vi "Param Global.vi"(7 "Operate":T2=enum."Read", 8 "error in (no error)":errorcluster caption="Error In", 9 "Param In":T1={"RH(%)"={"DS"={"阳极露点温度_DS"="TIRC101_PV", "阳极出口温度_DS"="TIR104_PV", "阴极露点温度_DS"="TIRC301_PV", "阴极出口温度_DS"="TIRC301_PV", "阳极相对湿度_DS"="SY_RH_An", "阴极相对湿度_DS"="SY_RH_Ca", "阳极露点温度设置_DS"="TIRC101_PV", "阳极出口温度设置_DS"="TIR104_PV", "阴极露点温度设置_DS"="TIRC301_PV", "阴极出口温度设置_DS"="TIRC301_PV"}, "Value"={"阳极露点温度_PV"=0.0, "阳极出口温度_PV"=0.0, "阴极露点温度_PV"=0.0, "阴极出口温度_PV"=0.0, "阳极相对湿度_SY"=0.0, "阴极相对湿度_SY"=0.0, "阳极露点温度设置_SV"=0.0, "阳极出口温度设置_SV"=0.0, "阴极露点温度设置_SV"=0.0, "阴极出口温度设置_SV"=0.0}}, "WEB"={"DS"={"自动模式(M0A1)_DS"="AUTO_MODE", "设备运行_DS"="DEVICE_STATE", "工步号_DS"="DEVICE_STATE", "运行模式_DS"="DEVICE_STATE"}, "Value"={"自动模式(M0A1)_PV"=FALSE, "设备运行_PV"=FALSE, "工步号_PV"=0.0, "运行模式_PV"=FALSE}}, "ELD"={"DS"={"负载电压设置_DS"="EL_V_SET", "负载电流设置_DS"="EL_A_SET", "负载功率设置_DS"="EL_P_SET", "负载模式设置_DS"="EL_MODE", "错误代码_DS"="EL_ERROR", "负载电压_DS"="EL_V", "负载电流_DS"="EL_A", "负载功率_DS"="EL_P", "负载输出使能_DS"="EL_INPUT", "负载连接_DS"="ELD", "负载升压_DS"="SY_Load_Rise_Volt", "负载升流_DS"="SY_Load_Rise_Curr", "负载升功率_DS"="SY_Load_Rise_Power", "负载降压_DS"="SY_Load_Drop_Volt", "负载降流_DS"="SY_Load_Drop_Curr", "负载降功率_DS"="SY_Load_Drop_Power", "电流密度_DS"="Density_A_SV", "功率密度_DS"="Density_P_SV"}, "Value"={"负载电压设置_SV"=0.0, "负载电流设置_SV"=0.0, "负载功率设置_SV"=0.0, "负载模式设置_SV"="", "错误代码_PV"="", "负载电压_PV"=0.0, "负载电流_PV"=0.0, "负载功率_PV"=0.0, "负载输出使能_SV"=FALSE, "负载连接_SY"=FALSE, "负载升压_SV"=0.0, "负载升流_SV"=0.0, "负载升功率_SV"=0.0, "负载降压_SV"=0.0, "负载降流_SV"=0.0, "负载降功率_SV"=0.0, "电流密度_SV"=0.0, "功率密度_SV"=0.0}}, "SY"={"DS"={"总报警_DS"="SY_Totol_Warning", "WEB连接_DS"="SY_Web_Con", "计量比功能_DS"="SY_Measurung_Ratio", "PLC连接_DS"="SY_Measurung_Ratio", "H2计量比功能_DS"="SY_Measurung_Ratio", "Air计量比功能_DS"="SY_Measurung_Ratio", "PLC失联报警_DS"="SY_Measurung_Ratio"}, "Value"={"总报警_PV"=FALSE, "WEB连接_PV"=FALSE, "计量比功能_SV"=FALSE, "PLC连接_SV"=FALSE, "H2计量比功能_SV"=FALSE, "Air计量比功能_SV"=FALSE, "PLC失联报警_SV"=FALSE}}, "PLC"={"DS"={"PLC急停_DS"="HMI_Estop_SV", "PLC连接_DS"="PLC", "下位机心跳值_DS"="PLC", "上位机心跳值_DS"="HMI_AlarmWord_SV", "上位机报警等级字_DS"="HMI_AlarmWord_SV", "负载可卸载_DS"="HMI_AlarmWord_SV"}, "Value"={"PLC急停_PV"=FALSE, "PLC连接_PV"=FALSE, "下位机心跳值_PV"=0.0, "上位机心跳值_SV"=0.0, "上位机报警等级字_SV"=0.0, "负载可卸载_SV"=FALSE}}, "Bool Control"={"DS"={"维护模式_DS"="WorkMode_SV", "阳极氮气吹扫_DS"="An_Purge_SV", "阴极氮气吹扫_DS"="Ca_Purge_SV", "阳极脉冲使能_DS"="An_Pulse_EN_SV", "准备好使能_DS"="DEVICE_READY", "阳极干湿气切换_DS"="An_GasMode_SV", "阴极干湿气切换_DS"="Ca_GasMode_SV", "自动/手动模式_DS"="AUTO_MODE", "入口背压_DS"="Stack_PreMode_SV", "手动卸载_DS"="HMI_Stack_OFF_SV", "软急停_DS"="HMI_Estop_SV", "负载连接_DS"="ELoad_EN_SV", "PLC故障复位_DS"="PLC_Alarm_Reset_SV", "蜂鸣器屏蔽_DS"="BuzzerShield_SV"}, "Value"={"维护模式_SV"=FALSE, "阳极氮气吹扫_SV"=FALSE, "阴极氮气吹扫_SV"=FALSE, "阳极脉冲使能_SV"=FALSE, "准备好使能_SV"=FALSE, "阳极干湿气切换_SV"=FALSE, "阴极干湿气切换_SV"=FALSE, "自动/手动模式_SV"=FALSE, "入口背压_SV"=FALSE, "手动卸载_SV"=FALSE, "软急停_SV"=FALSE, "负载连接_SV"=FALSE, "PLC故障复位_SV"=FALSE, "蜂鸣器屏蔽_SV"=FALSE}}, "Stoich"={"DS"={"H2初始流量_DS"="SY_Activation_Area", "Ait初始流量_DS"="SY_Pieces", "H2侧系数_DS"="SY_Activation_Area", "Air侧系数_DS"="SY_Pieces", "H2计量比_DS"="SY_Stoich_H2", "Air计量比_DS"="SY_Stoich_Air", "时间间隔_DS"="SY_Stoich_Interval", "H2计算气量_DS"="SY_Stoich_H2Flow", "Air计算气量_DS"="SY_Stoich_AirFlow", "H2流量_DS"="SY_Stoich_H2Flow", "Air流量_DS"="SY_Stoich_AirFlow"}, "Value"={"H2初始流量_SV"=0.0, "Ait初始流量_SV"=0.0, "H2侧系数_SV"=0.0, "Air侧系数_SV"=0.0, "H2计量比_SV"=0.0, "Air计量比_SV"=0.0, "时间间隔_SV"=0.0, "H2计算气量_SV"=0.0, "Air计算气量_SV"=0.0, "H2流量_DS"=0.0, "Air流量_DS"=0.0}}, "PLC Need"=[{"Name"="电堆电流_SV", "Identifier"="Stack_I_A_SV", "Source"="EL_A", "Value"=""}], "CVM"={"DS"={"活化面积_DS"="SY_Activation_Area", "开路电压_DS"="SY_OCV_Value", "单体总片数_DS"="SY_Pieces", "单体显示片数_DS"="SY_Pieces_Dis", "起始编号_DS"="SY_Starting_Number", "最大值"="SY_Activation_Area", "最大值编号_DS"="SY_OCV_Value", "最小值_DS"="SY_Pieces", "最小值编号_DS"="SY_Pieces_Dis", "选区合计电压_DS"="SY_Starting_Number", "平均值_DS"="SY_Pieces_Dis", "离均差_DS"="SY_Starting_Number"}, "Value"={"活化面积_SV"=0.0, "开路电压_SV"=0.0, "单体片数_SV"=0.0, "单体显示片数_SV"=0.0, "起始编号_SV"=0.0, "最大值_SV"=0.0, "最大值编号_SV"=0.0, "最小值_SV"=0.0, "最小值编号_SV"=0.0, "选区合计电压_SV"=0.0, "平均值_SV"=0.0, "离均差_SV"=0.0}}}, 11 "Project":string) -> (0 "error out":errorcluster caption="Error Out", 3 "Param Out":T1={"RH(%)"={"DS"={"阳极露点温度_DS"="TIRC101_PV", "阳极出口温度_DS"="TIR104_PV", "阴极露点温度_DS"="TIRC301_PV", "阴极出口温度_DS"="TIRC301_PV", "阳极相对湿度_DS"="SY_RH_An", "阴极相对湿度_DS"="SY_RH_Ca", "阳极露点温度设置_DS"="TIRC101_PV", "阳极出口温度设置_DS"="TIR104_PV", "阴极露点温度设置_DS"="TIRC301_PV", "阴极出口温度设置_DS"="TIRC301_PV"}, "Value"={"阳极露点温度_PV"=0.0, "阳极出口温度_PV"=0.0, "阴极露点温度_PV"=0.0, "阴极出口温度_PV"=0.0, "阳极相对湿度_SY"=0.0, "阴极相对湿度_SY"=0.0, "阳极露点温度设置_SV"=0.0, "阳极出口温度设置_SV"=0.0, "阴极露点温度设置_SV"=0.0, "阴极出口温度设置_SV"=0.0}}, "WEB"={"DS"={"自动模式(M0A1)_DS"="AUTO_MODE", "设备运行_DS"="DEVICE_STATE", "工步号_DS"="DEVICE_STATE", "运行模式_DS"="DEVICE_STATE"}, "Value"={"自动模式(M0A1)_PV"=FALSE, "设备运行_PV"=FALSE, "工步号_PV"=0.0, "运行模式_PV"=FALSE}}, "ELD"={"DS"={"负载电压设置_DS"="EL_V_SET", "负载电流设置_DS"="EL_A_SET", "负载功率设置_DS"="EL_P_SET", "负载模式设置_DS"="EL_MODE", "错误代码_DS"="EL_ERROR", "负载电压_DS"="EL_V", "负载电流_DS"="EL_A", "负载功率_DS"="EL_P", "负载输出使能_DS"="EL_INPUT", "负载连接_DS"="ELD", "负载升压_DS"="SY_Load_Rise_Volt", "负载升流_DS"="SY_Load_Rise_Curr", "负载升功率_DS"="SY_Load_Rise_Power", "负载降压_DS"="SY_Load_Drop_Volt", "负载降流_DS"="SY_Load_Drop_Curr", "负载降功率_DS"="SY_Load_Drop_Power", "电流密度_DS"="Density_A_SV", "功率密度_DS"="Density_P_SV"}, "Value"={"负载电压设置_SV"=0.0, "负载电流设置_SV"=0.0, "负载功率设置_SV"=0.0, "负载模式设置_SV"="", "错误代码_PV"="", "负载电压_PV"=0.0, "负载电流_PV"=0.0, "负载功率_PV"=0.0, "负载输出使能_SV"=FALSE, "负载连接_SY"=FALSE, "负载升压_SV"=0.0, "负载升流_SV"=0.0, "负载升功率_SV"=0.0, "负载降压_SV"=0.0, "负载降流_SV"=0.0, "负载降功率_SV"=0.0, "电流密度_SV"=0.0, "功率密度_SV"=0.0}}, "SY"={"DS"={"总报警_DS"="SY_Totol_Warning", "WEB连接_DS"="SY_Web_Con", "计量比功能_DS"="SY_Measurung_Ratio", "PLC连接_DS"="SY_Measurung_Ratio", "H2计量比功能_DS"="SY_Measurung_Ratio", "Air计量比功能_DS"="SY_Measurung_Ratio", "PLC失联报警_DS"="SY_Measurung_Ratio"}, "Value"={"总报警_PV"=FALSE, "WEB连接_PV"=FALSE, "计量比功能_SV"=FALSE, "PLC连接_SV"=FALSE, "H2计量比功能_SV"=FALSE, "Air计量比功能_SV"=FALSE, "PLC失联报警_SV"=FALSE}}, "PLC"={"DS"={"PLC急停_DS"="HMI_Estop_SV", "PLC连接_DS"="PLC", "下位机心跳值_DS"="PLC", "上位机心跳值_DS"="HMI_AlarmWord_SV", "上位机报警等级字_DS"="HMI_AlarmWord_SV", "负载可卸载_DS"="HMI_AlarmWord_SV"}, "Value"={"PLC急停_PV"=FALSE, "PLC连接_PV"=FALSE, "下位机心跳值_PV"=0.0, "上位机心跳值_SV"=0.0, "上位机报警等级字_SV"=0.0, "负载可卸载_SV"=FALSE}}, "Bool Control"={"DS"={"维护模式_DS"="WorkMode_SV", "阳极氮气吹扫_DS"="An_Purge_SV", "阴极氮气吹扫_DS"="Ca_Purge_SV", "阳极脉冲使能_DS"="An_Pulse_EN_SV", "准备好使能_DS"="DEVICE_READY", "阳极干湿气切换_DS"="An_GasMode_SV", "阴极干湿气切换_DS"="Ca_GasMode_SV", "自动/手动模式_DS"="AUTO_MODE", "入口背压_DS"="Stack_PreMode_SV", "手动卸载_DS"="HMI_Stack_OFF_SV", "软急停_DS"="HMI_Estop_SV", "负载连接_DS"="ELoad_EN_SV", "PLC故障复位_DS"="PLC_Alarm_Reset_SV", "蜂鸣器屏蔽_DS"="BuzzerShield_SV"}, "Value"={"维护模式_SV"=FALSE, "阳极氮气吹扫_SV"=FALSE, "阴极氮气吹扫_SV"=FALSE, "阳极脉冲使能_SV"=FALSE, "准备好使能_SV"=FALSE, "阳极干湿气切换_SV"=FALSE, "阴极干湿气切换_SV"=FALSE, "自动/手动模式_SV"=FALSE, "入口背压_SV"=FALSE, "手动卸载_SV"=FALSE, "软急停_SV"=FALSE, "负载连接_SV"=FALSE, "PLC故障复位_SV"=FALSE, "蜂鸣器屏蔽_SV"=FALSE}}, "Stoich"={"DS"={"H2初始流量_DS"="SY_Activation_Area", "Ait初始流量_DS"="SY_Pieces", "H2侧系数_DS"="SY_Activation_Area", "Air侧系数_DS"="SY_Pieces", "H2计量比_DS"="SY_Stoich_H2", "Air计量比_DS"="SY_Stoich_Air", "时间间隔_DS"="SY_Stoich_Interval", "H2计算气量_DS"="SY_Stoich_H2Flow", "Air计算气量_DS"="SY_Stoich_AirFlow", "H2流量_DS"="SY_Stoich_H2Flow", "Air流量_DS"="SY_Stoich_AirFlow"}, "Value"={"H2初始流量_SV"=0.0, "Ait初始流量_SV"=0.0, "H2侧系数_SV"=0.0, "Air侧系数_SV"=0.0, "H2计量比_SV"=0.0, "Air计量比_SV"=0.0, "时间间隔_SV"=0.0, "H2计算气量_SV"=0.0, "Air计算气量_SV"=0.0, "H2流量_DS"=0.0, "Air流量_DS"=0.0}}, "PLC Need"=[{"Name"="电堆电流_SV", "Identifier"="Stack_I_A_SV", "Source"="EL_A", "Value"=""}], "CVM"={"DS"={"活化面积_DS"="SY_Activation_Area", "开路电压_DS"="SY_OCV_Value", "单体总片数_DS"="SY_Pieces", "单体显示片数_DS"="SY_Pieces_Dis", "起始编号_DS"="SY_Starting_Number", "最大值"="SY_Activation_Area", "最大值编号_DS"="SY_OCV_Value", "最小值_DS"="SY_Pieces", "最小值编号_DS"="SY_Pieces_Dis", "选区合计电压_DS"="SY_Starting_Number", "平均值_DS"="SY_Pieces_Dis", "离均差_DS"="SY_Starting_Number"}, "Value"={"活化面积_SV"=0.0, "开路电压_SV"=0.0, "单体片数_SV"=0.0, "单体显示片数_SV"=0.0, "起始编号_SV"=0.0, "最大值_SV"=0.0, "最大值编号_SV"=0.0, "最小值_SV"=0.0, "最小值编号_SV"=0.0, "选区合计电压_SV"=0.0, "平均值_SV"=0.0, "离均差_SV"=0.0}}})   [LabVIEW 2020]
uses:
  Data Global/Data Global Mode.ctl
  0007 Controls/SY_Parameter.ctl
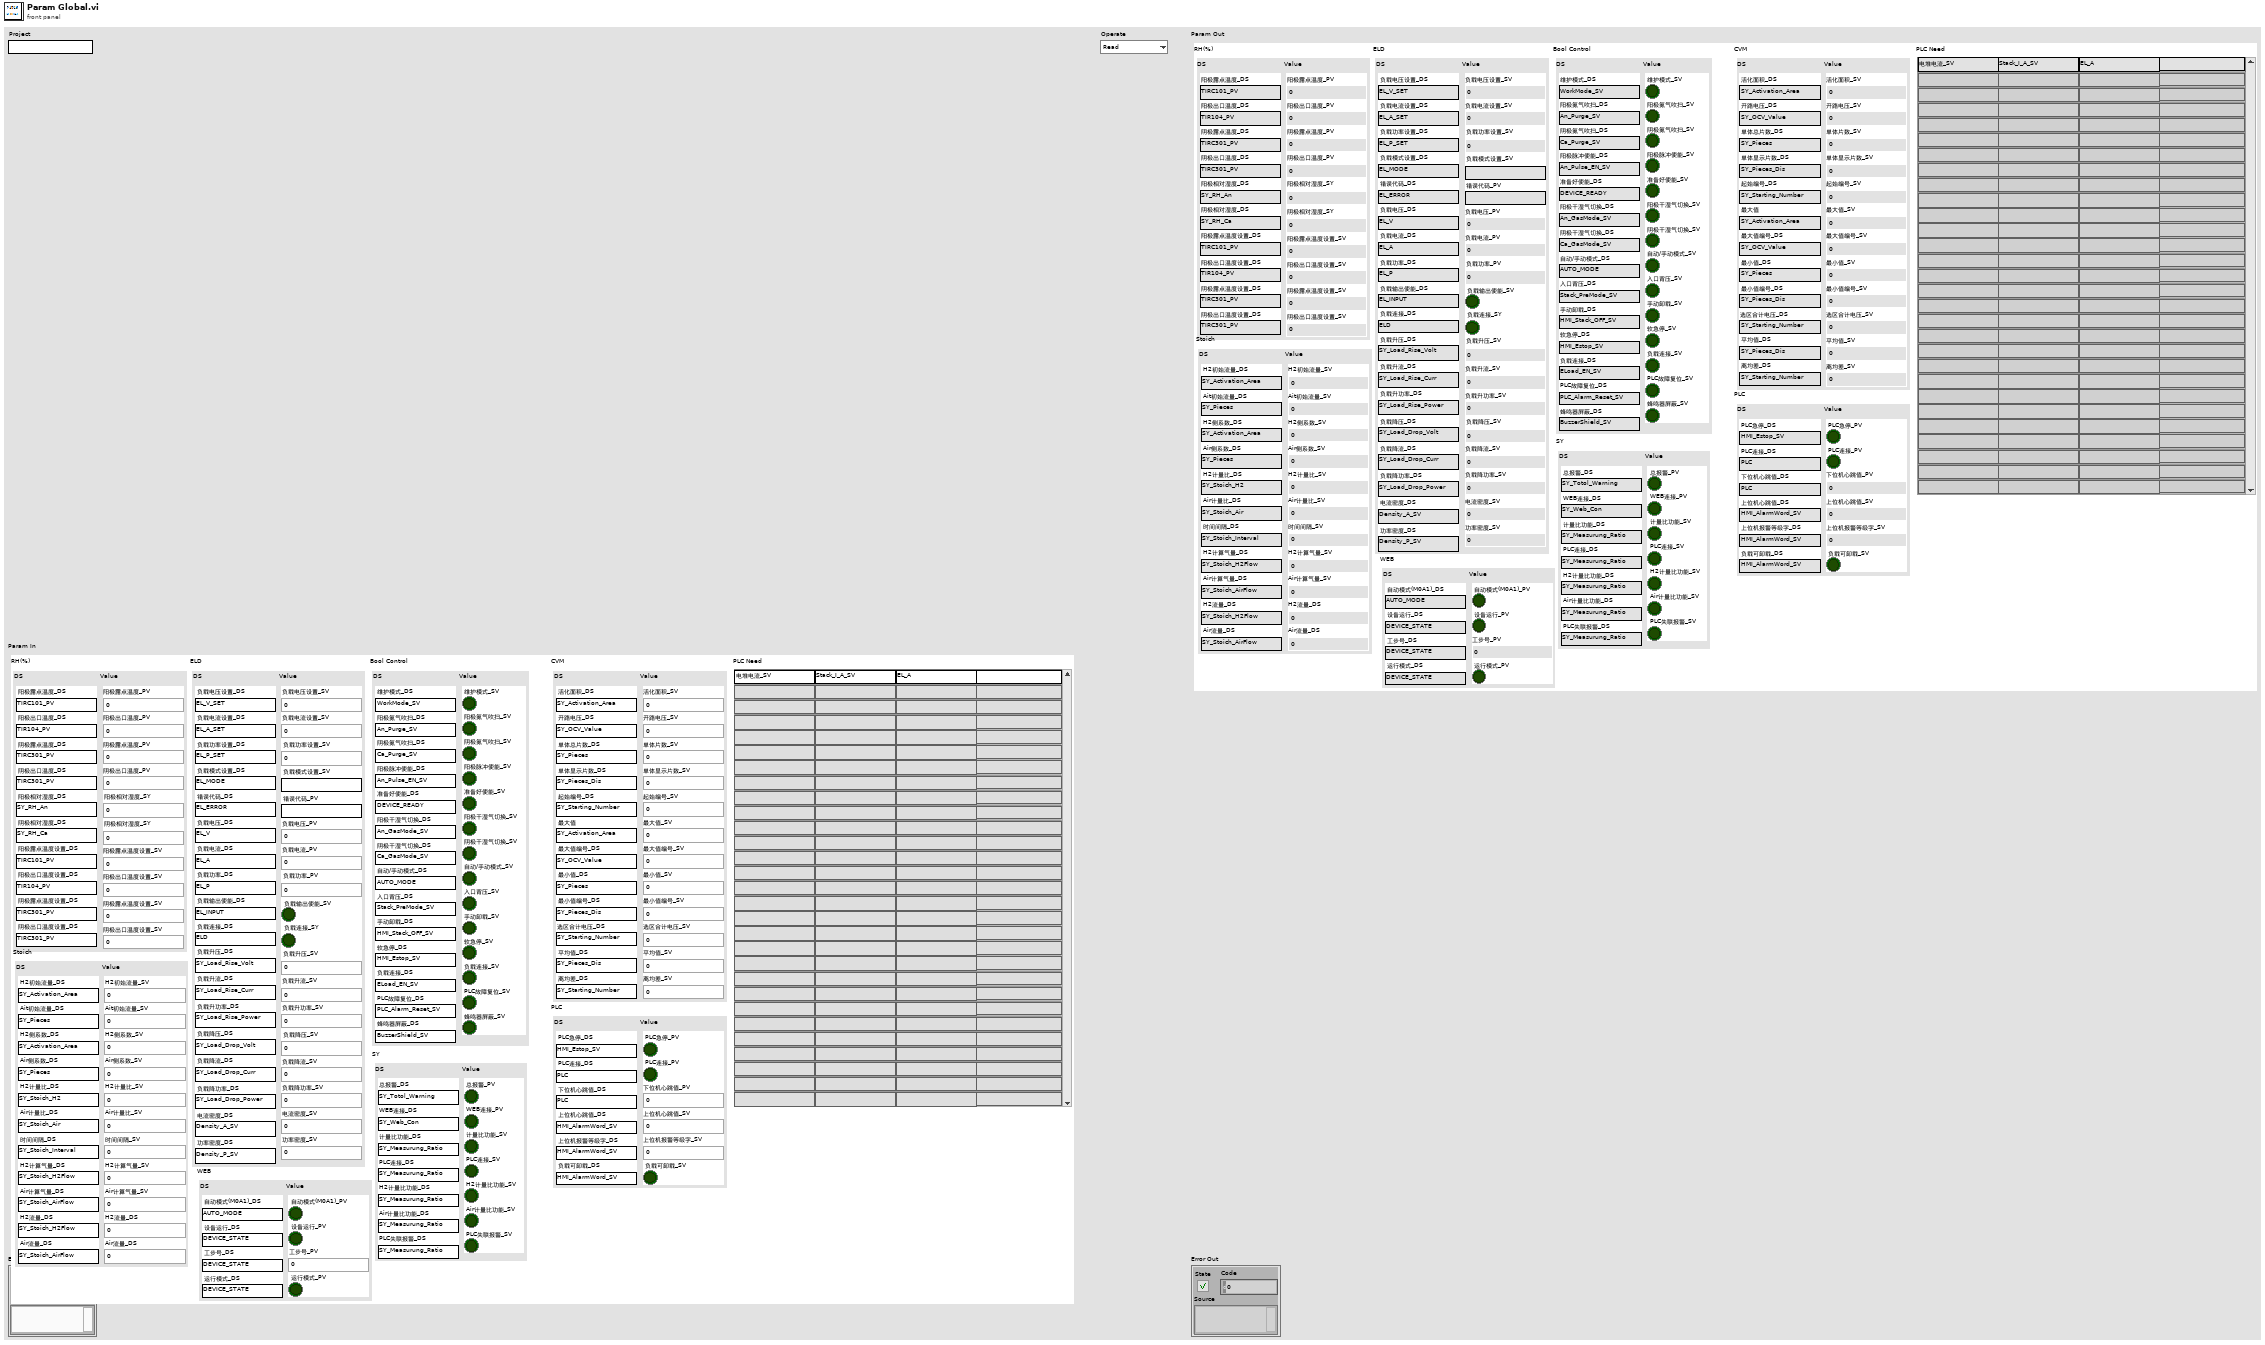
[diagram p1: front panel]
types:
  T1 = typedef "SY_Parameter.ctl" = cluster{"RH(%)":cluster{"DS":cluster{"阳极露点温度_DS":string, "阳极出口温度_DS":string, "阴极露点温度_DS":string, "阴极出口温度_DS":string, "阳极相对湿度_DS":string, "阴极相对湿度_DS":string, "阳极露点温度设置_DS":string, "阳极出口温度设置_DS":string, "阴极露点温度设置_DS":string, "阴极出口温度设置_DS":string}, "Value":cluster{"阳极露点温度_PV":sgl, "阳极出口温度_PV":sgl, "阴极露点温度_PV":sgl, "阴极出口温度_PV":sgl, "阳极相对湿度_SY":sgl, "阴极相对湿度_SY":sgl, "阳极露点温度设置_SV":sgl, "阳极出口温度设置_SV":sgl, "阴极露点温度设置_SV":sgl, "阴极出口温度设置_SV":sgl}}, "WEB":cluster{"DS":cluster{"自动模式(M0A1)_DS":string, "设备运行_DS":string, "工步号_DS":string, "运行模式_DS":string}, "Value":cluster{"自动模式(M0A1)_PV":bool, "设备运行_PV":bool, "工步号_PV":sgl, "运行模式_PV":bool}}, "ELD":cluster{"DS":cluster{"负载电压设置_DS":string, "负载电流设置_DS":string, "负载功率设置_DS":string, "负载模式设置_DS":string, "错误代码_DS":string, "负载电压_DS":string, "负载电流_DS":string, "负载功率_DS":string, "负载输出使能_DS":string, "负载连接_DS":string, "负载升压_DS":string, "负载升流_DS":string, "负载升功率_DS":string, "负载降压_DS":string, "负载降流_DS":string, "负载降功率_DS":string, "电流密度_DS":string, "功率密度_DS":string}, "Value":cluster{"负载电压设置_SV":sgl, "负载电流设置_SV":sgl, "负载功率设置_SV":sgl, "负载模式设置_SV":string, "错误代码_PV":string, "负载电压_PV":sgl, "负载电流_PV":sgl, "负载功率_PV":sgl, "负载输出使能_SV":bool, "负载连接_SY":bool, "负载升压_SV":sgl, "负载升流_SV":sgl, "负载升功率_SV":sgl, "负载降压_SV":sgl, "负载降流_SV":sgl, "负载降功率_SV":sgl, "电流密度_SV":sgl, "功率密度_SV":sgl}}, "SY":cluster{"DS":cluster{"总报警_DS":string, "WEB连接_DS":string, "计量比功能_DS":string, "PLC连接_DS":string, "H2计量比功能_DS":string, "Air计量比功能_DS":string, "PLC失联报警_DS":string}, "Value":cluster{"总报警_PV":bool, "WEB连接_PV":bool, "计量比功能_SV":bool, "PLC连接_SV":bool, "H2计量比功能_SV":bool, "Air计量比功能_SV":bool, "PLC失联报警_SV":bool}}, "PLC":cluster{"DS":cluster{"PLC急停_DS":string, "PLC连接_DS":string, "下位机心跳值_DS":string, "上位机心跳值_DS":string, "上位机报警等级字_DS":string, "负载可卸载_DS":string}, "Value":cluster{"PLC急停_PV":bool, "PLC连接_PV":bool, "下位机心跳值_PV":sgl, "上位机心跳值_SV":sgl, "上位机报警等级字_SV":sgl, "负载可卸载_SV":bool}}, "Bool Control":cluster{"DS":cluster{"维护模式_DS":string, "阳极氮气吹扫_DS":string, "阴极氮气吹扫_DS":string, "阳极脉冲使能_DS":string, "准备好使能_DS":string, "阳极干湿气切换_DS":string, "阴极干湿气切换_DS":string, "自动/手动模式_DS":string, "入口背压_DS":string, "手动卸载_DS":string, "软急停_DS":string, "负载连接_DS":string, "PLC故障复位_DS":string, "蜂鸣器屏蔽_DS":string}, "Value":cluster{"维护模式_SV":bool, "阳极氮气吹扫_SV":bool, "阴极氮气吹扫_SV":bool, "阳极脉冲使能_SV":bool, "准备好使能_SV":bool, "阳极干湿气切换_SV":bool, "阴极干湿气切换_SV":bool, "自动/手动模式_SV":bool, "入口背压_SV":bool, "手动卸载_SV":bool, "软急停_SV":bool, "负载连接_SV":bool, "PLC故障复位_SV":bool, "蜂鸣器屏蔽_SV":bool}}, "Stoich":cluster{"DS":cluster{"H2初始流量_DS":string, "Ait初始流量_DS":string, "H2侧系数_DS":string, "Air侧系数_DS":string, "H2计量比_DS":string, "Air计量比_DS":string, "时间间隔_DS":string, "H2计算气量_DS":string, "Air计算气量_DS":string, "H2流量_DS":string, "Air流量_DS":string}, "Value":cluster{"H2初始流量_SV":sgl, "Ait初始流量_SV":sgl, "H2侧系数_SV":sgl, "Air侧系数_SV":sgl, "H2计量比_SV":sgl, "Air计量比_SV":sgl, "时间间隔_SV":sgl, "H2计算气量_SV":sgl, "Air计算气量_SV":sgl, "H2流量_DS":sgl, "Air流量_DS":sgl}}, "PLC Need":cluster{"Name":string, "Identifier":string, "Source":string, "Value":string}[], "CVM":cluster{"DS":cluster{"活化面积_DS":string, "开路电压_DS":string, "单体总片数_DS":string, "单体显示片数_DS":string, "起始编号_DS":string, "最大值":string, "最大值编号_DS":string, "最小值_DS":string, "最小值编号_DS":string, "选区合计电压_DS":string, "平均值_DS":string, "离均差_DS":string}, "Value":cluster{"活化面积_SV":sgl, "开路电压_SV":sgl, "单体片数_SV":sgl, "单体显示片数_SV":sgl, "起始编号_SV":sgl, "最大值_SV":sgl, "最大值编号_SV":sgl, "最小值_SV":sgl, "最小值编号_SV":sgl, "选区合计电压_SV":sgl, "平均值_SV":sgl, "离均差_SV":sgl}}}
  T2 = typedef "Data Global Mode.ctl" = enum16{"Init", "Read", "Write", "Write Data", "Load"}
  T3 = typedef "SDQ Data Type.ctl" = cluster{"CAN Length":string, "CAN Name":string, "CAN ID":string, "CAN Type":string, "Test Item":string, "Byte Order":string, "Instruction":string, "Control Type":string, "Group":string, "Offset":dbl, "Coefficient":dbl, "Write Enable":bool, "Lable Type":string, "Key?":string, "Set Value":string, "Upper":dbl, "Lower":dbl, "Unit":string, "Formula":string, "Test Item Type":string, "Length":i32, "Address":string, "Name":string, "Identifier":string, "Data Type":string, "Enumerate?":string, "Enumerate List":string, "Data":string, "Source":string}
  T4 = cluster{"Name":string, "Identifier":string, "Source":string, "Value":string}[]
  T5 = cluster{"Name":string, "Identifier":string, "Source":string, "Value":string}
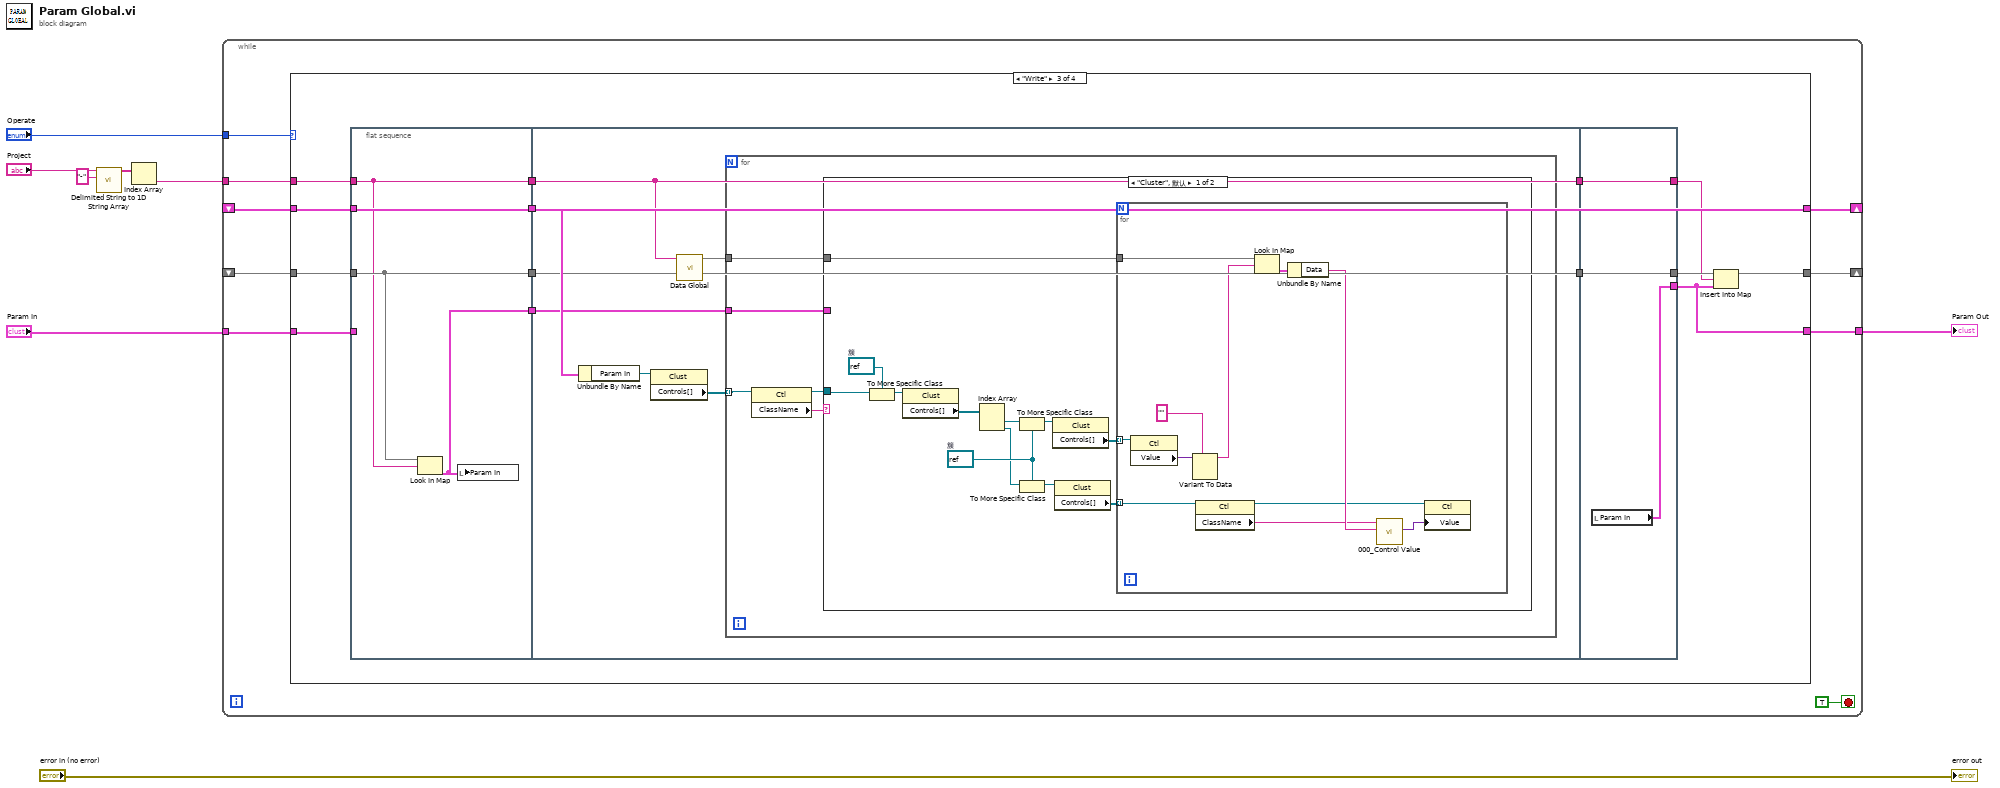
[diagram p0: block diagram]
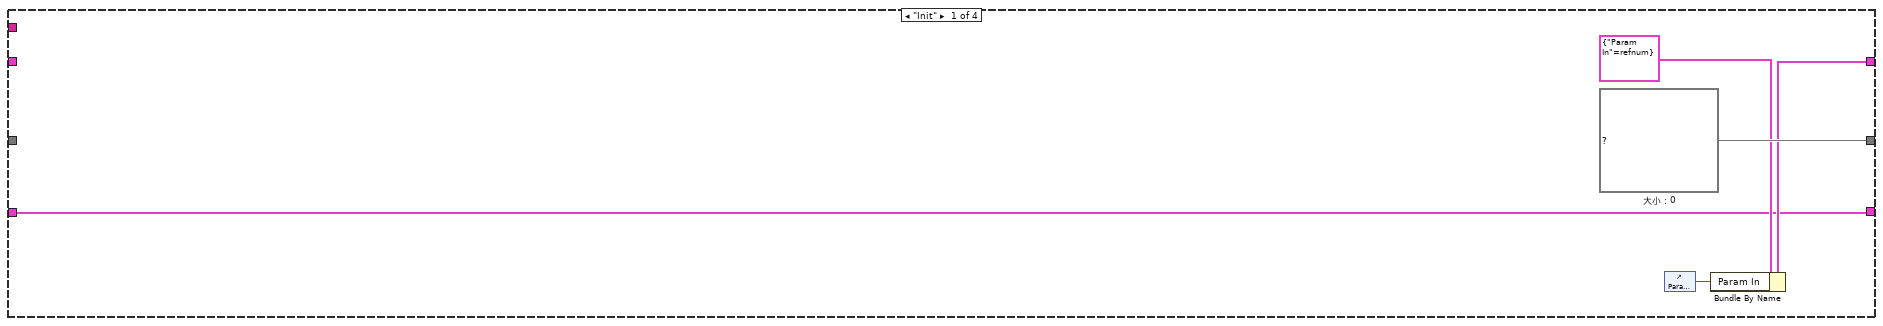
[diagram p2: hidden frame]
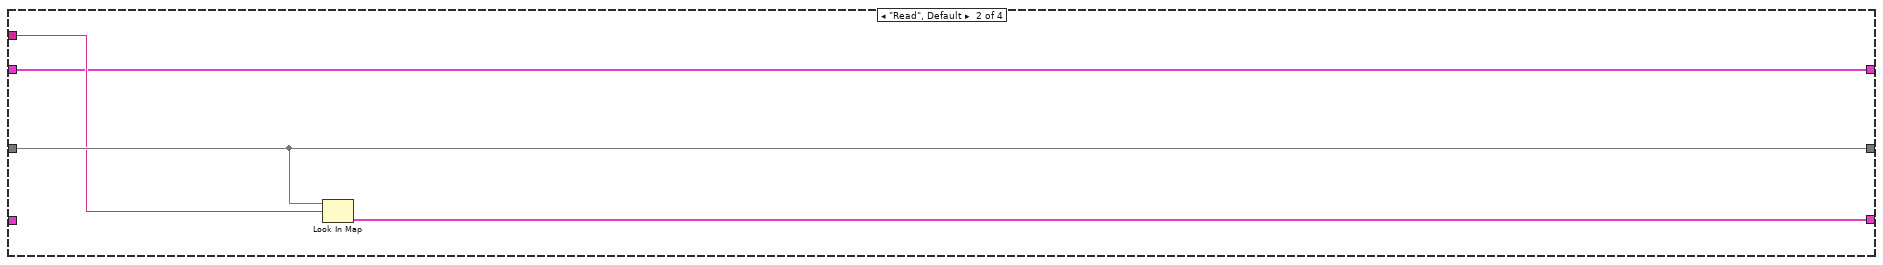
[diagram p3: hidden frame]
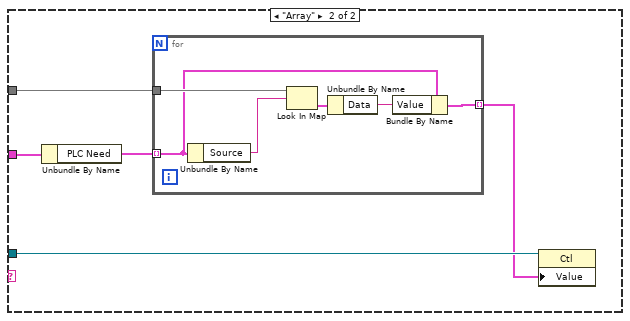
[diagram p4: hidden frame]
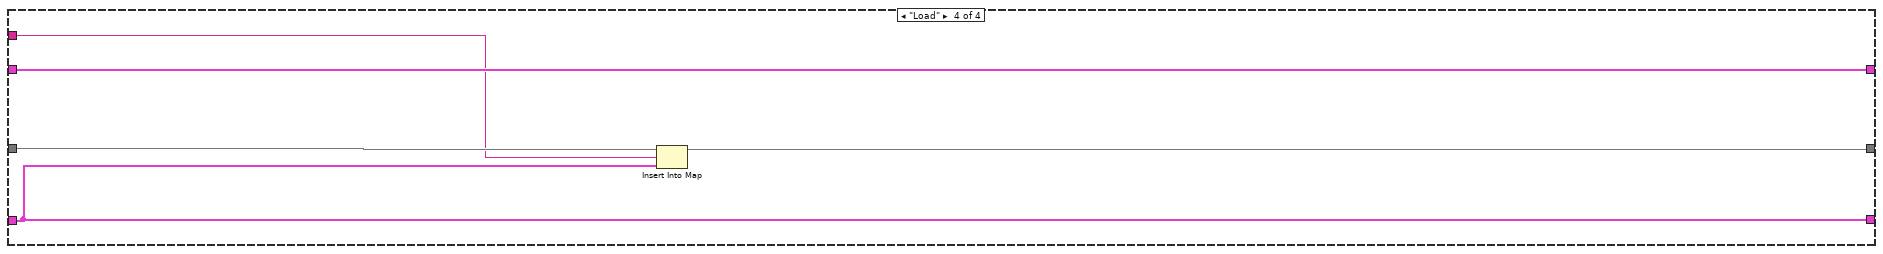
[diagram p5: hidden frame]
diagram:
  n1 = call <vilib>:"Delimited String to 1D String Array.vi"("delimiter"="-", "delimited string"="Project") -> ("string array"=w3:string[])  [unwired: 9 in]
  n2 = Index Array(array=w3) -> (element=w1:string)  [unwired: 1 in]
  n3 = while {
    tunnel: "Operate" -> [w16]
    tunnel: w1 -> [w15]
    shift-right: [w17] -> _
    shift-left: _ -> [w14]
    tunnel: [w12] -> w6
    shift-right: [w11] -> _
    shift-left: _ -> [w10]
    tunnel: "Param In" -> [w9]
    stop <- TRUE stop-if-true
    n4 = case shown="\"Write\"" w16 {
      tunnel: [w22 w26 w39 w95] -> w17
      tunnel: w15 -> [_ w25 w37 w96]
      tunnel: w14 -> [_ w26 w36 w97]
      tunnel: [w18 w24 w27 w94] -> w12
      tunnel: [w19 w23 w40 w98] -> w11
      tunnel: w10 -> [_ w23 w40 w98]
      tunnel: w9 -> [w18 _ w29 w94]
      frame "Init" {
        w22 = map{string, T1} {}  # 大小：0
        n5 = control-ref of="Param In"() -> (w20:refnum<vi>)
        n6 = Bundle By Name(cluster=cluster{"Param In":refnum<vi>} {"Param In"=refnum}, "Param In"=w20) -> (w19:cluster{"Param In":refnum<vi>})
      }
      frame "Read", Default {
        n7 = Look In Map(map=w26, key=w25) -> (value=w24:T1)  [unwired: 1 in, 1 out]
      }
      frame "Write" {
        n8 = flat-sequence {
          tunnel: w40 -> [w44]
          tunnel: [w44] -> w38
          tunnel: w37 -> [w42]
          tunnel: w36 -> [w43]
          tunnel: [w43] -> w35
          tunnel: [w42] -> w30
          tunnel: w29 -> [_]
          tunnel: [w41] -> w28
          tunnel: w38 -> [w51]
          tunnel: w35 -> [w48]
          tunnel: [w48] -> w34
          tunnel: [w46] -> w31
          tunnel: w30 -> [w46]
          tunnel: w28 -> [w47]
          tunnel: [w93] -> w33
          tunnel: w34 -> [w93]
          tunnel: [w92] -> w32
          tunnel: w31 -> [w92]
          tunnel: [w91] -> w27
          frame #0 {
            n9 = Look In Map(map=w43, key=w42) -> (value=w41:T1)  [unwired: 1 in, 1 out]
            n10 = local write "Param In"(w41) -> ()
          }
          frame #1 {
            n11 = Unbundle By Name(w51) -> ("Param In"=w50:refnum<vi>)
            n12 = property class="Clust"(reference=w50) -> ("Controls[]"=w49:refnum<vi>[])  [unwired: 1 in, 2 out]
            n13 = call "Data Global.vi"("Name"=w46) -> ("Data Out"=w45:map{string, T3})  [unwired: 7 in, 3 out]
            n14 = for {
              tunnel: w49 -> [w56] mode=indexing
              tunnel: w45 -> [w53]
              tunnel: w47 -> [w52]
              n15 = property class="Ctl"(reference=w56) -> (reference out=w54:refnum<vi>, "ClassName"=w55:string)  [unwired: 1 in, 1 out]
              n16 = case shown="\"Cluster\", 默认" w55 {
                tunnel: w54 -> [w68 w81]
                tunnel: w53 -> [w58 w82]
                tunnel: w52 -> [_ w84]
                frame "Cluster", Default {
                  w60 = refnum<vi> refnum  # 簇
                  w67 = refnum<vi> refnum  # 簇
                  n17 = To More Specific Class(target class=w67, reference=w68) -> (specific class reference=w66:refnum<vi>)  [unwired: 1 in, 1 out]
                  n18 = property class="Clust"(reference=w66) -> ("Controls[]"=w65:refnum<vi>[])  [unwired: 1 in, 2 out]
                  n19 = Index Array(array=w65) -> (element #1=w61:refnum<vi>, element #2=w57:refnum<vi>)  [unwired: 2 in]
                  n20 = To More Specific Class(target class=w60, reference=w61) -> (specific class reference=w64:refnum<vi>)  [unwired: 1 in, 1 out]
                  n21 = To More Specific Class(target class=w60, reference=w57) -> (specific class reference=w62:refnum<vi>)  [unwired: 1 in, 1 out]
                  n22 = property class="Clust"(reference=w64) -> ("Controls[]"=w63:refnum<vi>[])  [unwired: 1 in, 2 out]
                  n23 = property class="Clust"(reference=w62) -> ("Controls[]"=w59:refnum<vi>[])  [unwired: 1 in, 2 out]
                  n24 = for {
                    tunnel: w63 -> [w79] mode=indexing
                    tunnel: w59 -> [w72] mode=indexing
                    tunnel: w58 -> [w76]
                    n25 = property class="Ctl"(reference=w79) -> ("Value"=w78:variant)  [unwired: 1 in, 2 out]
                    n26 = Variant To Data(type="", Variant=w78) -> (data=w75:string)  [unwired: 1 in, 1 out]
                    n27 = property class="Ctl"(reference=w72) -> (reference out=w70:refnum<vi>, "ClassName"=w71:string)  [unwired: 1 in, 1 out]
                    n28 = Look In Map(map=w76, key=w75) -> (value=w74:T3)  [unwired: 1 in, 1 out]
                    n29 = Unbundle By Name(w74) -> ("Data"=w73:string)
                    n30 = call "000_Control Value.vi"("Value String In"=w73, "Class Name"=w71) -> ("Value Out"=w69:variant)  [unwired: 8 in, 1 out]
                    n31 = property class="Ctl"(reference=w70, "Value"=w69) -> ()  [unwired: 1 in, 2 out]
                  }
                }
                frame "Array" {
                  n32 = Unbundle By Name(w84) -> ("PLC Need"=w83:T4)
                  n33 = for {
                    tunnel: w83 -> [w87] mode=indexing
                    tunnel: w82 -> [w89]
                    tunnel: [w85] -> w80 mode=indexing
                    n34 = Unbundle By Name(w87) -> ("Source"=w88:string)
                    n35 = Look In Map(map=w89, key=w88) -> (value=w90:T3)  [unwired: 1 in, 1 out]
                    n36 = Unbundle By Name(w90) -> ("Data"=w86:string)
                    n37 = Bundle By Name(cluster=w87, "Value"=w86) -> (w85:T5)
                  }
                  n38 = property class="Ctl"(reference=w81, "Value"=w80) -> ()  [unwired: 1 in, 2 out]
                }
              }
            }
          }
          frame #2 {
            n39 = local read "Param In"() -> (w91:T1)
          }
        }
        n40 = Insert Into Map(map in=w33, key=w32, value=w27) -> (map out=w39:map{string, T1})  [unwired: 2 out]
      }
      frame "Load" {
        n41 = Insert Into Map(map in=w97, key=w96, value=w94) -> (map out=w95:map{string, T1})  [unwired: 2 out]
      }
    }
  }
  "Param Out" <- w6
  "error out" <- "error in (no error)"
